vi "RWA_Extract Section from File String.vi"(9 "Section Name":string, 11 "String":string) -> (2 "Found? Out":bool, 3 "String Out":string)   [LabVIEW 2023]
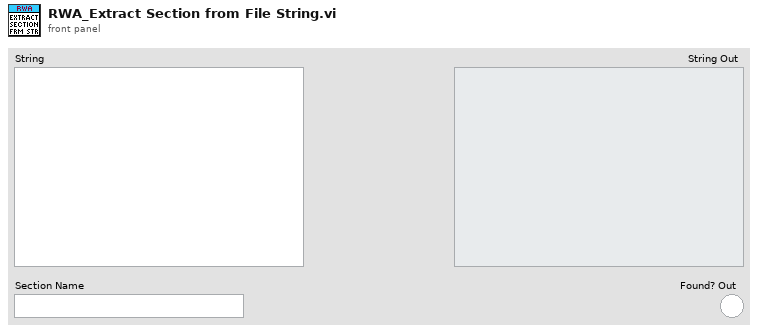
[diagram p1: front panel]
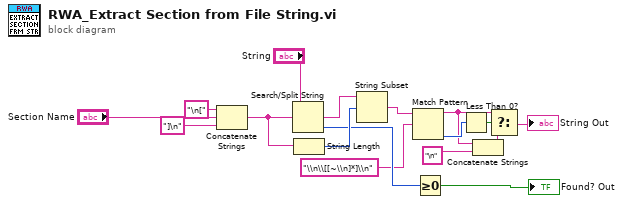
[diagram p0: block diagram]
diagram:
  n1 = Concatenate Strings("\n[" ("string"), "Section Name", "]\n" ("string")) -> (w10:string)
  n2 = Search/Split String(string="String", search string/char (-)=w10) -> (match + rest of string=w8:string, offset of match=w6:i32)  [unwired: 1 in, 1 out]
  n3 = String Length(string=w10) -> (length=w11:i32)
  n4 = String Subset(string=w8, offset (0)=w11) -> (substring=w9:string)  [unwired: 1 in]
  n5 = Match Pattern(string=w9, regular expression="\\n\\[[~\\n]*]\\n") -> (before substring=w14:string, offset past match=w16:i32)  [unwired: 3 out]
  n6 = Greater Or Equal To 0?(x=w6) -> (x >= 0?=→"Found? Out":bool)
  n7 = Less Than 0?(x=w16) -> (x < 0?=w17:bool)
  n8 = Concatenate Strings(w14, "\n" ("string")) -> (w13:string)
  n9 = Select(t=w14, s=w17, f=w13) -> (s? t:f=→"String Out":string)
